vi "GetMasterInfo.vi"(4 "数据in":string) -> (0 "主站信息":T1 {"时间戳" format="%016x"; "帧号" format="%04x"; "主站IP" format="%08x"}, 1 "cyclicInfo":i32)   [LabVIEW 2018]
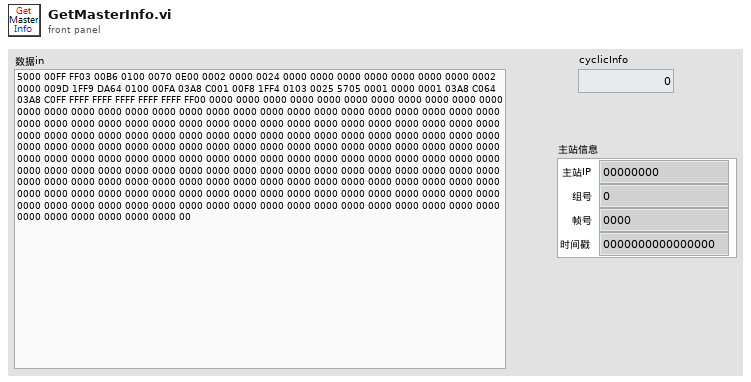
[diagram p1: front panel]
types:
  T1 = cluster{"主站IP":u32, "组号":u8, "帧号":u16, "时间戳":u64}
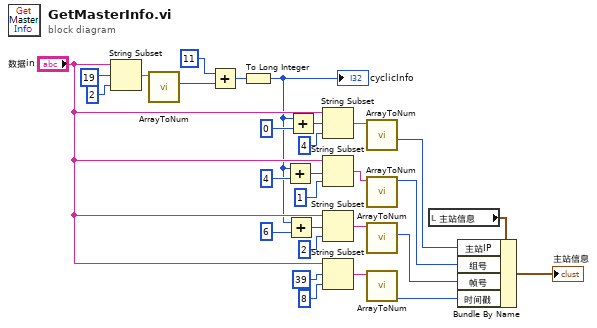
[diagram p0: block diagram]
diagram:
  n1 = String Subset(string="数据in", offset (0)=19 ("长度（剩余）"), length (rest)=2 ("偏移量(0)")) -> (substring=w27:string)
  n2 = call "ArrayToNum.vi"("输入字符串"=w27) -> ("2B"=w26:u16)  [unwired: 3 in, 3 out]
  n3 = Add(x=u16 11, y=w26) -> (x+y=w6:u16)
  n4 = To Long Integer(number=w6) -> (32bit integer=w1:i32)
  "cyclicInfo" <- w1
  n5 = Add(x=w1, y=4 ("索引")) -> (x+y=w5:i32)
  n6 = Add(x=w1, y=6 ("索引")) -> (x+y=w3:i32)
  n7 = Add(x=w1, y=0 ("索引")) -> (x+y=w8:i32)
  n8 = String Subset(string="数据in", offset (0)=w8, length (rest)=4 ("长度")) -> (substring=w24:string)
  n9 = String Subset(string="数据in", offset (0)=w5, length (rest)=1 ("长度")) -> (substring=w23:string)
  n10 = String Subset(string="数据in", offset (0)=w3, length (rest)=2 ("长度")) -> (substring=w22:string)
  n11 = String Subset(string="数据in", offset (0)=39 ("索引"), length (rest)=8 ("长度")) -> (substring=w21:string)
  n12 = call "ArrayToNum.vi"("输入字符串"=w24) -> ("4B"=w19:u32)  [unwired: 3 in, 3 out]
  n13 = call "ArrayToNum.vi"("输入字符串"=w23) -> ("1B"=w18:u8)  [unwired: 3 in, 3 out]
  n14 = call "ArrayToNum.vi"("输入字符串"=w22) -> ("2B"=w17:u16)  [unwired: 3 in, 3 out]
  n15 = call "ArrayToNum.vi"("输入字符串"=w21) -> ("8B"=w16:u64)  [unwired: 3 in, 3 out]
  n16 = local read "主站信息"() -> (w20:T1)
  n17 = Bundle By Name(cluster=w20, "主站IP"=w19, "组号"=w18, "帧号"=w17, "时间戳"=w16) -> (→"主站信息":T1)
